vi "Set Duty Cycle.vi"(7 "error in (no error)":errorcluster, 9 "Duty Cycle":dbl=0.5, 10 "PWM Ref In":T1) -> (0 "error out":errorcluster, 3 "PWM Ref Out":T1)   [LabVIEW 2021, in "PWM.lvlib"]
doc: "Sets the duty cycle value of a pulse width modulation (PWM) signal."
uses:
  <vilib>/myRIO/Instrument Drivers/Onboard IO/PWM/PWM.lvlib
  <vilib>/myRIO/Instrument Drivers/Onboard IO/PWM/typedefs/PWM Reference.ctl
  <vilib>/myRIO/Common/Instrument Driver Framework/Utilities/typedefs/myRIO Generic Hardware Reference.ctl
  <vilib>/myRIO/Common/Instrument Driver Framework/Utilities/typedefs/Hardware Version Enum.ctl
  <vilib>/myRIO/Common/Instrument Driver Framework/Utilities/typedefs/myRIO v1.0 Reference.ctl
  <vilib>/myRIO/Common/Instrument Driver Framework/Utilities/typedefs/Generic FPGA Reference.ctl
  <vilib>/myRIO/Common/Instrument Driver Framework/myRIO v1.0/PWM/typedefs/PWM Channels Enum.ctl
  <vilib>/myRIO/Instrument Drivers/Onboard IO/PWM/typedefs/PWM Configuration.ctl
  <vilib>/myRIO/Common/Instrument Driver Framework/myRIO v1.0/PWM/vis/myRIO v1.0 Write PWM.vi
  <vilib>/myRIO/Common/Instrument Driver Framework/roboRIO v1.0/PWM/vis/roboRIO v1.0 Write PWM.vi
  <vilib>/myRIO/Common/Instrument Driver Framework/ELVIS III v1.0/PWM/vis/ELVIS III v1.0 Write PWM.vi
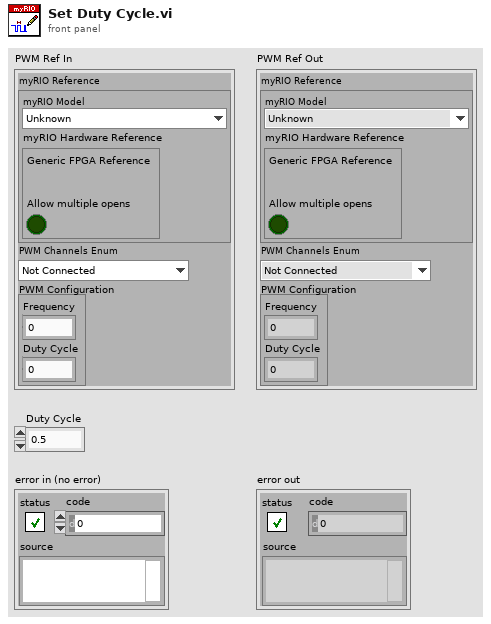
[diagram p1: front panel]
types:
  T1 = typedef "PWM.lvlib/PWM Reference.ctl" = cluster{"myRIO Reference":T2, "PWM Channels Enum":T6, "PWM Configuration":T7}
  T2 = typedef "myRIO Generic Hardware Reference.ctl" = cluster{"myRIO Model":T3, "myRIO Hardware Reference":T4}
  T3 = typedef "Hardware Version Enum.ctl" = enum16{"Unknown", "myRIO-1900", "myRIO-1950", "roboRIO", "NI ELVIS RIO CM", "ELVIS III"}
  T4 = typedef "myRIO v1.0 Reference.ctl" = cluster{"Generic FPGA Reference":T5, "Allow multiple opens":bool}
  T5 = typedef "Generic FPGA Reference.ctl" = refnum<k20>
  T6 = typedef "PWM Channels Enum.ctl" = enum16{"Not Connected", "C/PWM0", "C/PWM1", "A/PWM0", "A/PWM1", "A/PWM2", "A/PWM3", "A/PWM4", "A/PWM5", "A/PWM6", "A/PWM7", "A/PWM8", "A/PWM9", "A/PWM10", "A/PWM11", "A/PWM12", "A/PWM13", "A/PWM14", "A/PWM15", "A/PWM16", "A/PWM17", "A/PWM18", "A/PWM19", "B/PWM0", "B/PWM1", "B/PWM2", "B/PWM3", "B/PWM4", "B/PWM5", "B/PWM6", "B/PWM7", "B/PWM8", "B/PWM9", "B/PWM10", "B/PWM11", "B/PWM12", "B/PWM13", "B/PWM14", "B/PWM15", "B/PWM16", "B/PWM17", "B/PWM18", "B/PWM19", "PWM/PWM0", "PWM/PWM1", "PWM/PWM2", "PWM/PWM3", "PWM/PWM4", "PWM/PWM5", "PWM/PWM6", "PWM/PWM7", "PWM/PWM8", "PWM/PWM9"}
  T7 = typedef "PWM.lvlib/PWM Configuration.ctl" = cluster{"Frequency":dbl, "Duty Cycle":dbl}
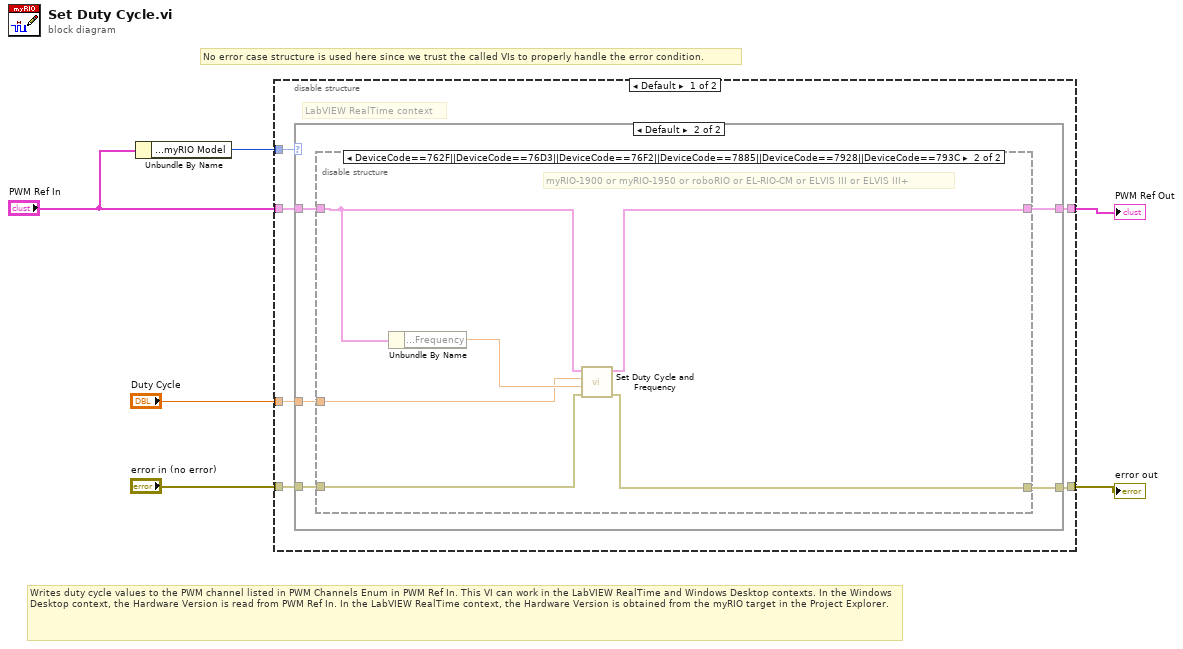
[diagram p0: block diagram]
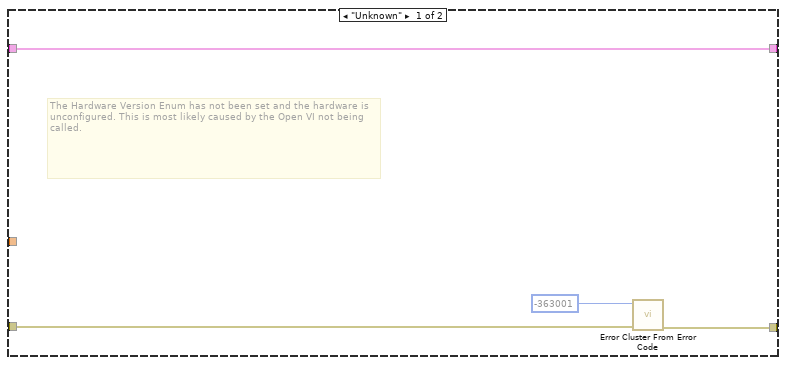
[diagram p2: hidden frame]
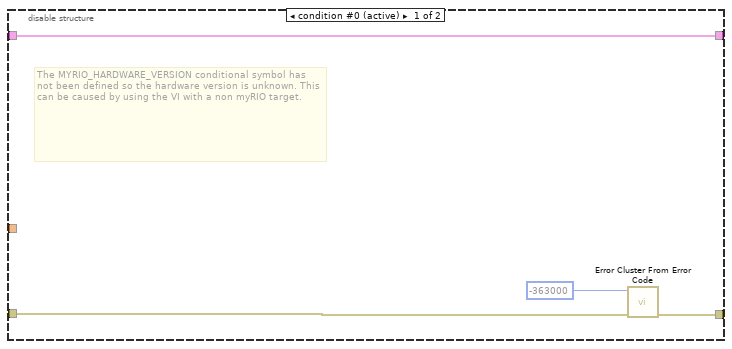
[diagram p3: hidden frame]
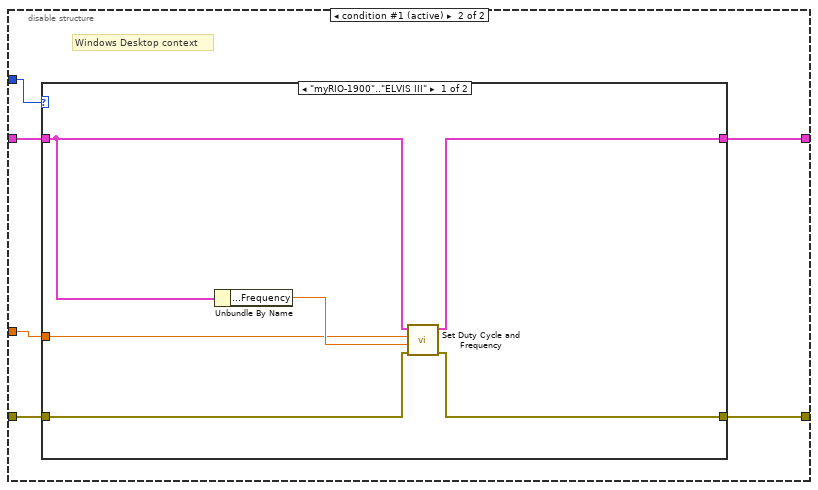
[diagram p4: hidden frame]
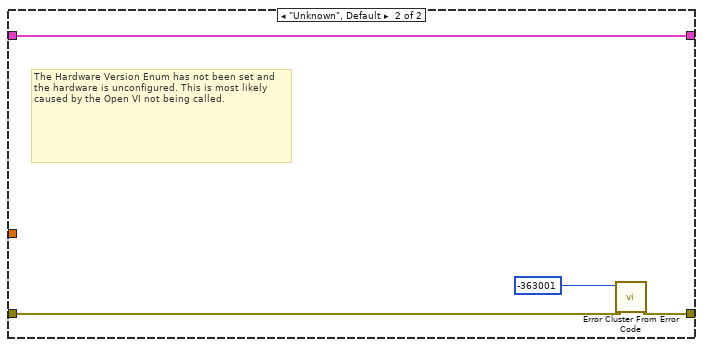
[diagram p5: hidden frame]
diagram:
  # "No error case structure is used here since we trust the called VIs to properly handle the error condition."
  # "Writes duty cycle values to the PWM channel listed in PWM Channels Enum in PWM Ref In. This VI can work in the LabVIEW RealTime and Windows Desktop contexts. In the Windows Desktop context, the Hardware Version is read from PWM Ref In. In the LabVIEW RealTime context, the Hardware Version is obtained from the myRIO target in the Project Explorer."
  n1 = Unbundle By Name("PWM Ref In") -> ("myRIO Reference.myRIO Model"=w2:T3)
  n2 = disable-structure shown="Default" {
    disable-tunnel: [w12 w37] -> w3
    disable-tunnel: "PWM Ref In" -> [w11 w34]
    disable-tunnel: "error in (no error)" -> [w10 w36]
    disable-tunnel: [w9 w35] -> w4
    disable-tunnel: w2 -> [w8 w33]
    disable-tunnel: "Duty Cycle" -> [w7 w32]
    frame condition #0 {
      # "LabVIEW RealTime context"
      n3 = case shown="Default" w8 {
        tunnel: [w15 w21] -> w12
        tunnel: w11 -> [w13 w20]
        tunnel: w10 -> [w14 w19]
        tunnel: [w13 w18] -> w9
        tunnel: w7 -> [_ w17]
        frame "Unknown" {
          # "The Hardware Version Enum has not been set and the hardware is unconfigured. This is most likely caused by the Open VI not being called."
          n4 = call <vilib>:"Error Cluster From Error Code.vi"("error in (no error)"=w14, "error code (0)"=-363001) -> ("error out"=w15:errorcluster)  [unwired: 7 in]
        }
        frame Default {
          n5 = disable-structure shown="DeviceCode==762F||DeviceCode==76D3||DeviceCode==76F2||DeviceCode==7885||DeviceCode==7928||DeviceCode==793C" {
            disable-tunnel: w20 -> [w22 w31]
            disable-tunnel: [w25 w26] -> w21
            disable-tunnel: w19 -> [w23 w27]
            disable-tunnel: [w22 w28] -> w18
            disable-tunnel: w17 -> [_ w29]
            frame condition #0 (active) {
              # "The MYRIO_HARDWARE_VERSION conditional symbol has not been defined so the hardware version is unknown. This can be caused by using the VI with a non myRIO target."
              n6 = call <vilib>:"Error Cluster From Error Code.vi"("error in (no error)"=w23, "error code (0)"=-363000) -> ("error out"=w25:errorcluster)  [unwired: 7 in]
            }
            frame condition #1 {
              # "myRIO-1900 or myRIO-1950 or roboRIO or EL-RIO-CM or ELVIS III or ELVIS III+"
              n7 = Unbundle By Name(w31) -> ("PWM Configuration.Frequency"=w30:dbl)
              n8 = call <vilib>:"Set Duty Cycle and Frequency.vi"("error in (no error)"=w27, "Frequency [Hz]"=w30, "Duty Cycle"=w29, "PWM Ref In"=w31) -> ("error out"=w26:errorcluster, "PWM Ref Out"=w28:T1)  [unwired: 5 in]
            }
          }
        }
      }
    }
    frame condition #1 (active) {
      # "Windows Desktop context"
      n9 = case shown="\"myRIO-1900\"..\"ELVIS III\"" w33 {
        tunnel: [w38 w47] -> w37
        tunnel: w34 -> [w42 w44]
        tunnel: w36 -> [w39 w45]
        tunnel: [w41 w44] -> w35
        tunnel: w32 -> [w40 _]
        frame "myRIO-1900".."ELVIS III" {
          n10 = Unbundle By Name(w42) -> ("PWM Configuration.Frequency"=w43:dbl)
          n11 = call <vilib>:"Set Duty Cycle and Frequency.vi"("error in (no error)"=w39, "Frequency [Hz]"=w43, "Duty Cycle"=w40, "PWM Ref In"=w42) -> ("error out"=w38:errorcluster, "PWM Ref Out"=w41:T1)  [unwired: 5 in]
        }
        frame "Unknown", Default {
          # "The Hardware Version Enum has not been set and the hardware is unconfigured. This is most likely caused by the Open VI not being called."
          n12 = call <vilib>:"Error Cluster From Error Code.vi"("error in (no error)"=w45, "error code (0)"=-363001) -> ("error out"=w47:errorcluster)  [unwired: 7 in]
        }
      }
    }
  }
  "PWM Ref Out" <- w4
  "error out" <- w3
